vi "Reduce WFRM.vi"(6 "decimation factor":i32, 7 "Decimation method":T1(ring)=enum."Min-Max", 8 "error in (no error)":errorcluster, 11 "Waveform":waveform(sgl)) -> (0 "error out":errorcluster, 3 "Waveform out":waveform(sgl))   [LabVIEW 2015]
uses:
  <vilib>/measure/maresamp.llb/Resample Waveform (single shot).vi
  <vilib>/measure/NI_MAPro.lvlib
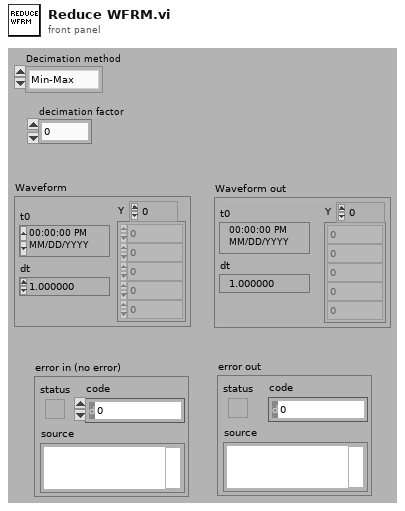
[diagram p1: front panel]
types:
  T1 = enum16{"coerce", "linear", "spline", "Min-Max", "Average"}
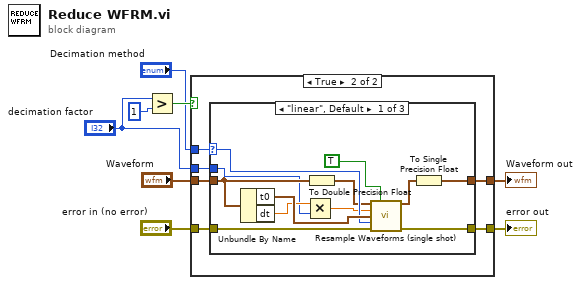
[diagram p0: block diagram]
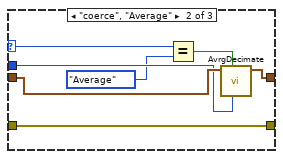
[diagram p3: hidden frame]
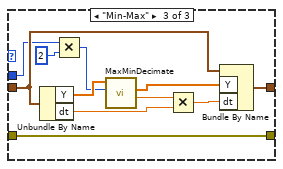
[diagram p4: hidden frame]
diagram:
  n1 = Greater?(x="decimation factor", y=1) -> (0:w8:bool)
  n2 = case shown="True" w8 {
    tunnel: [w10 w16] -> w2
    tunnel: "Decimation method" -> [_ w15]
    tunnel: [w9 w14] -> w4
    tunnel: "error in (no error)" -> [w9 w13]
    tunnel: "Waveform" -> [w10 w12]
    tunnel: "decimation factor" -> [_ w11]
    frame False {
    }
    frame True {
      n3 = case shown="\"linear\", Default" w15 {
        selector: w15 -> [w26 w30 _]
        tunnel: w12 -> [w27 w35 w45]
        tunnel: w11 -> [w22 w33 w43]
        tunnel: [w17 w34 w42] -> w16
        tunnel: [w25 w32 w38] -> w14
        tunnel: w13 -> [w24 w32 w38]
        frame "linear", Default {
          n4 = Unbundle By Name(w27) -> ("t0"=w28:timestamp, "dt"=w23:dbl)
          n5 = Multiply(x=w23, y=w22) -> (x*y=w21:dbl)
          n6 = To Double Precision Float(number=w27) -> (double precision float=w20:waveform(dbl))
          n7 = call-poly <vilib>:"Resample Waveforms (single shot).vi"("waveform in"=w20, "open interval? (F)"=TRUE, "dt"=w21, "t0"=w28, "interpolation mode"=w26, "error in (no error)"=w24) -> ("resampled waveform out"=w18:waveform(dbl), "error out"=w25:errorcluster)  [unwired: 1 in, 7 out]
          n8 = To Single Precision Float(number=w18) -> (single precision float=w17:waveform(sgl))
        }
        frame "coerce", "Average" {
          n9 = Equal?(x=w30, y=T1."Average" ("Plot interpolation")) -> (x = y?=w29:bool)
          n10 = call "AvrgDecimate.vi"("Decimate by"=w33, "Average?"=w29, "waveform"=w35) -> ("output waveform"=w34:waveform(sgl))  [unwired: 8 out]
        }
        frame "Min-Max" {
          n11 = Unbundle By Name(w45) -> ("Y"=w46:sgl[], "dt"=w39:dbl)
          n12 = Multiply(x=w43, y=2) -> (x*y=w37:i32)
          n13 = call "MaxMinDecimate.vi"("decimation factor"=w37, "Array"=w46) -> ("actual decimation"=w41:sgl, "decimated array"=w44:sgl[])  [unwired: 8 out]
          n14 = Multiply(x=w41, y=w39) -> (x*y=w40:dbl)
          n15 = Bundle By Name(cluster=w45, "Y"=w44, "dt"=w40) -> (w42:waveform(sgl))
        }
      }
    }
  }
  "error out" <- w4
  "Waveform out" <- w2
